vi "test metadata.vi"() -> (0 "ook":errorcluster, 1 "setgetok":bool, 2 "deletedok":bool, 3 "overwriteok":bool, 4 "error ok":bool)   [LabVIEW 2025, in "NISE_CEF_Tests.lvlib"]
uses:
  NISE_CEF_Tests.lvlib
  Trunk/Configuration Framework/serializable configuration/NISE_CEF_serializable configuration.lvclass
panel:
  out "error 538502":errorcluster
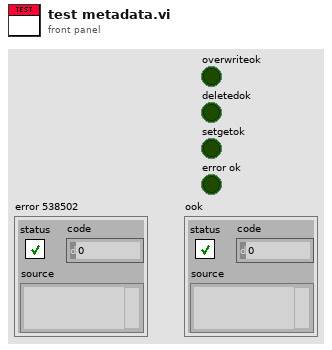
[diagram p1: front panel]
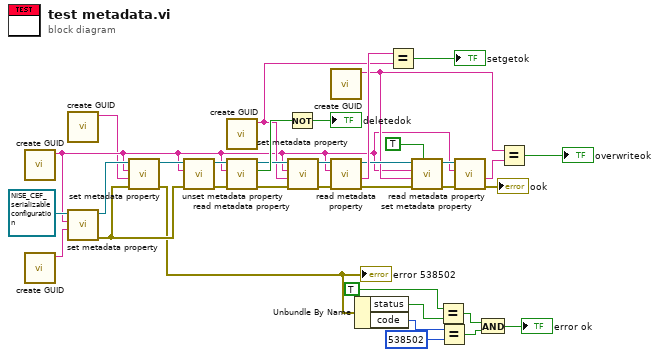
[diagram p0: block diagram]
diagram:
  n1 = call "create GUID.vi"() -> ("uuid"=w11:string)  [unwired: 10 in, 1 out]
  n2 = call "create GUID.vi"() -> ("uuid"=w10:string)  [unwired: 10 in, 1 out]
  n3 = call "create GUID.vi"() -> ("uuid"=w9:string)  [unwired: 10 in, 1 out]
  n4 = call "set metadata property.vi"("value"=w10, "key"=w11, "configuration in"=refnum<class "NISE_CEF_serializable configuration.lvclass"> refnum ("configuration")) -> ("error out"=w33:errorcluster, "configuration out"=w35:refnum<class "NISE_CEF_serializable configuration.lvclass">)  [unwired: 7 in]
  n5 = call "set metadata property.vi"("error in"=w33, "value"=w9, "key"=w11, "configuration in"=w35) -> ("error out"=w8:errorcluster, "configuration out"=w34:refnum<class "NISE_CEF_serializable configuration.lvclass">)  [unwired: 6 in]
  "error 538502" <- w8
  n6 = call "unset metadata property.vi"("error in"=w33, "key"=w11, "configuration in"=w34) -> ("error out"=w32:errorcluster, "configuration out"=w31:refnum<class "NISE_CEF_serializable configuration.lvclass">)  [unwired: 7 in]
  n7 = call "create GUID.vi"() -> ("uuid"=w24:string)  [unwired: 10 in, 1 out]
  n8 = call "read metadata property.vi"("error in"=w32, "key"=w11, "configuration in"=w31) -> ("error out"=w29:errorcluster, "found"=w30:bool, "configuration out"=w28:refnum<class "NISE_CEF_serializable configuration.lvclass">)  [unwired: 5 in, 1 out]
  n9 = Not(x=w30) -> (.not. x?=→"deletedok":bool)
  n10 = call "set metadata property.vi"("error in"=w29, "value"=w24, "key"=w11, "configuration in"=w28) -> ("error out"=w27:errorcluster, "configuration out"=w26:refnum<class "NISE_CEF_serializable configuration.lvclass">)  [unwired: 6 in]
  n11 = call "create GUID.vi"() -> ("uuid"=w12:string)  [unwired: 10 in, 1 out]
  n12 = call "read metadata property.vi"("error in"=w27, "key"=w11, "configuration in"=w26) -> ("error out"=w21:errorcluster, "value"=w25:string, "configuration out"=w20:refnum<class "NISE_CEF_serializable configuration.lvclass">)  [unwired: 5 in, 1 out]
  n13 = Unbundle By Name(w8) -> ("status"=w6:bool, "code"=w5:i32)
  n14 = Equal?(x=w25, y=w24) -> (x = y?=→"setgetok":bool)
  n15 = call "set metadata property.vi"("overwrite?"=TRUE, "error in"=w21, "value"=w12, "key"=w11, "configuration in"=w20) -> ("error out"=w17:errorcluster, "configuration out"=w18:refnum<class "NISE_CEF_serializable configuration.lvclass">)  [unwired: 5 in]
  n16 = Equal?(x=TRUE ("status"), y=w6) -> (x = y?=w3:bool)
  n17 = Equal?(x=w5, y=538502) -> (x = y?=w2:bool)
  n18 = call "read metadata property.vi"("error in"=w17, "key"=w11, "configuration in"=w18) -> ("error out"=→"ook":errorcluster, "value"=w15:string)  [unwired: 5 in, 2 out]
  n19 = And(x=w3, y=w2) -> (x .and. y?=→"error ok":bool)
  n20 = Equal?(x=w12, y=w15) -> (x = y?=→"overwriteok":bool)
